vi "Set value by string.vi"(8 "error in (no error)":errorcluster, 10 "Value":string, 11 "Column in":refnum<class "Composed Column.lvclass">) -> (0 "error out":errorcluster, 3 "Column out":refnum<class "Composed Column.lvclass">)   [LabVIEW 2020, in "Composed Columns.lvlib" / "Composed Column.lvclass"]
uses:
  Composed Column.lvclass
  Composed Column.lvclass/Composed Column.ctl
  Composed Columns/Value Source Interface Class/Value Source.lvclass
  Value Type/Value Type.lvclass
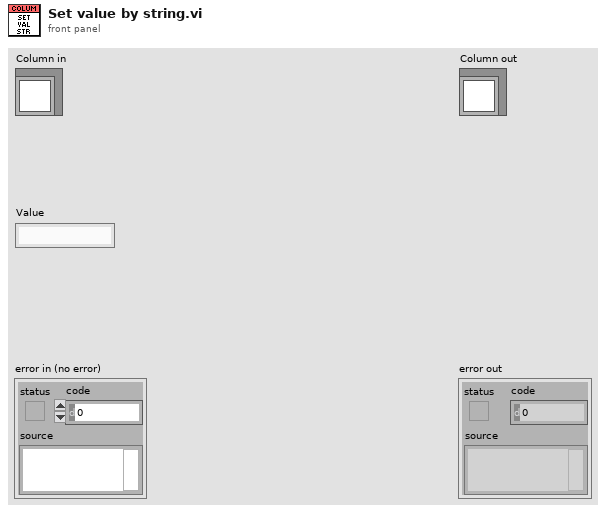
[diagram p1: front panel]
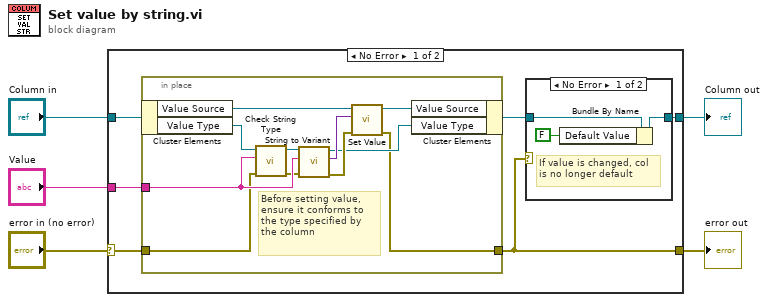
[diagram p0: block diagram]
diagram:
  n1 = case shown="No Error" "error in (no error)" {
    selector: "error in (no error)" -> [w10 w28]
    tunnel: [w8 w28] -> w4
    tunnel: "Column in" -> [w11 w27]
    tunnel: [w6 w27] -> w2
    tunnel: "Value" -> [w9 _]
    frame No Error {
      n2 = in-place {
        in-place-border: w10 -> [w20]
        in-place-border: w9 -> [w24]
        in-place-border: [w16] -> w8
        # "Before setting value, ensure it conforms to the type specified by the column"
        n3 = in-place-cluster #1(w11) -> ("Value Source"=w22:refnum<class "Value Source.lvclass">, "Value Type"=w26:refnum<class "Value Type.lvclass">)
        n4 = call-dynamic "Check String Type.vi"("error in (no error)"=w20, "String"=w24, "Value Type in"=w26) -> ("error out"=w19:errorcluster, "Value Type out"=w25:refnum<class "Value Type.lvclass">)  [unwired: 7 in]
        n5 = call-dynamic "String to Variant.vi"("error in (no error)"=w19, "String"=w24, "Value Type in"=w25) -> ("error out"=w18:errorcluster, "Variant"=w23:variant, "Value Type out"=w17:refnum<class "Value Type.lvclass">)  [unwired: 6 in]
        n6 = call-dynamic "Set Value.vi"("error in (no error)"=w18, "Variant"=w23, "Value Source in"=w22) -> ("error out"=w16:errorcluster, "Value Source out"=w21:refnum<class "Value Source.lvclass">)  [unwired: 7 in]
        n7 = in-place-cluster #1("Value Source"=w21, "Value Type"=w17) -> (w7:refnum<class "Composed Column.lvclass">)
      }
      n8 = case shown="No Error" w8 {
        tunnel: w7 -> [w14 w15]
        tunnel: [w13 w15] -> w6
        frame No Error {
          # "If value is changed, col\nis no longer default"
          n9 = Bundle By Name(cluster=w14, "Default Value"=FALSE) -> (w13:refnum<class "Composed Column.lvclass">)
        }
        frame Error {
        }
      }
    }
    frame Error {
    }
  }
  "error out" <- w4
  "Column out" <- w2
